vi "Text_for_latex.vi"(1 "Input String":string) -> (0 "Output String":string)   [LabVIEW 2012]
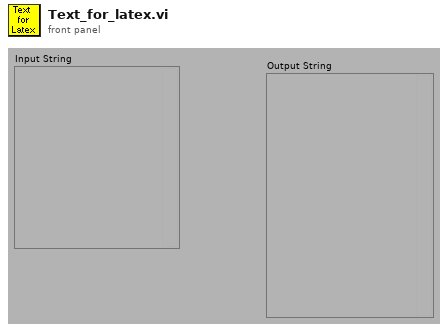
[diagram p1: front panel]
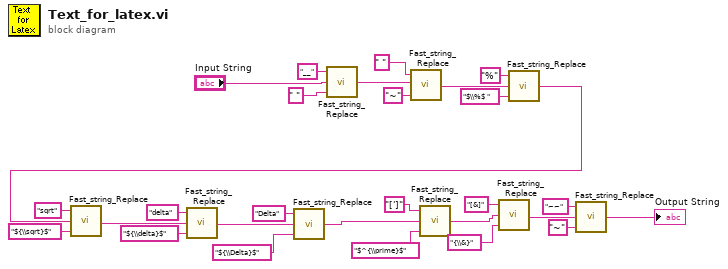
[diagram p0: block diagram]
diagram:
  n1 = call "Fast_string_Replace.vi"("Replace match with:"=" ", "Input String"="Input String", "regular expression"="__") -> ("Output String"=w2:string)  [unwired: 2 out]
  n2 = call "Fast_string_Replace.vi"("Replace match with:"="~", "Input String"=w2, "regular expression"=" ") -> ("Output String"=w13:string)  [unwired: 2 out]
  n3 = call "Fast_string_Replace.vi"("Replace match with:"="$\\%$ ", "Input String"=w13, "regular expression"="%") -> ("Output String"=w7:string)  [unwired: 2 out]
  n4 = call "Fast_string_Replace.vi"("Replace match with:"="${\\sqrt}$", "Input String"=w7, "regular expression"="sqrt") -> ("Output String"=w6:string)  [unwired: 2 out]
  n5 = call "Fast_string_Replace.vi"("Replace match with:"="${\\delta}$", "Input String"=w6, "regular expression"="delta") -> ("Output String"=w20:string)  [unwired: 2 out]
  n6 = call "Fast_string_Replace.vi"("Replace match with:"="${\\Delta}$", "Input String"=w20, "regular expression"="Delta") -> ("Output String"=w21:string)  [unwired: 2 out]
  n7 = call "Fast_string_Replace.vi"("Replace match with:"="$^{\\prime}$", "Input String"=w21, "regular expression"="[']") -> ("Output String"=w16:string)  [unwired: 2 out]
  n8 = call "Fast_string_Replace.vi"("Replace match with:"="{\\&}", "Input String"=w16, "regular expression"="[&]") -> ("Output String"=w10:string)  [unwired: 2 out]
  n9 = call "Fast_string_Replace.vi"("Replace match with:"="~", "Input String"=w10, "regular expression"="~~") -> ("Output String"=→"Output String":string)  [unwired: 2 out]
